vi "CMI Sync V3 Set Tigger.vi"(8 "error in":errorcluster, 9 "Trigger input logic (5V)":T1=enum."TTL 5V", 10 "Trigger mode (Auto)":T2=enum."Auto (continuous)", 11 "session in":T3={"VISA"="", "baud rate [bd/s]"=115200, "source"=enum."Auto", "hv range"=enum."1kV", "fsrc is fixed"=FALSE, "fsrc [Hz]"=10000000.0, "freq integ [s]"=1.0, "freq filter"=5, "trig level"=enum."TTL 5V", "chn1 mode"=enum."Source divider", "chn1 level"=enum."Positive 5V", "chn2 mode"=enum."Source divider", "chn2 level"=enum."Positive 5V", "chn2 div"=1, "chn3 mode"=enum."Chn 1 Active", "chn3 level"=enum."Positive 5V", "chn1 div entry"=enum."Calculate nearest divisor from measured fx", "chn1 dev limit [%]"=1.0, "chn1 check dev"=FALSE} {"chn2 div" min=1 max=100000000 step=1; "fsrc [Hz]" format="%_8p"}) -> (0 "error out":errorcluster, 3 "session out":T3={"VISA"="", "baud rate [bd/s]"=115200, "source"=enum."Auto", "hv range"=enum."1kV", "fsrc is fixed"=FALSE, "fsrc [Hz]"=10000000.0, "freq integ [s]"=1.0, "freq filter"=5, "trig level"=enum."TTL 5V", "chn1 mode"=enum."Source divider", "chn1 level"=enum."Positive 5V", "chn2 mode"=enum."Source divider", "chn2 level"=enum."Positive 5V", "chn2 div"=1, "chn3 mode"=enum."Chn 1 Active", "chn3 level"=enum."Positive 5V", "chn1 div entry"=enum."Calculate nearest divisor from measured fx", "chn1 dev limit [%]"=1.0, "chn1 check dev"=FALSE} {"chn2 div" min=1 max=100000000 step=1; "fsrc [Hz]" format="%_8p"})   [LabVIEW 2020, in "AWG.lvlib" / "CMI Sync Unit V3.lvlib"]
doc: "Sets trigger source and parameters."
uses:
  CMI Sync Unit V3.lvlib
  CMI Sync V3 session.ctl
  CMI Sync V3 Reference Clock Source.ctl
  CMI Sync V3 HV input Range.ctl
  CMI Sync V3 Trigger Input Level.ctl
  CMI Sync V3 Channel 1 Mode.ctl
  CMI Sync V3 Channel Output Levels.ctl
  CMI Sync V3 Channel 2 Mode.ctl
  CMI Sync V3 Channel 3 Mode.ctl
  CMI Sync V3 Channel 1 Divisor Entry Mode.ctl
  CMI Sync V3 Trigger Mode.ctl
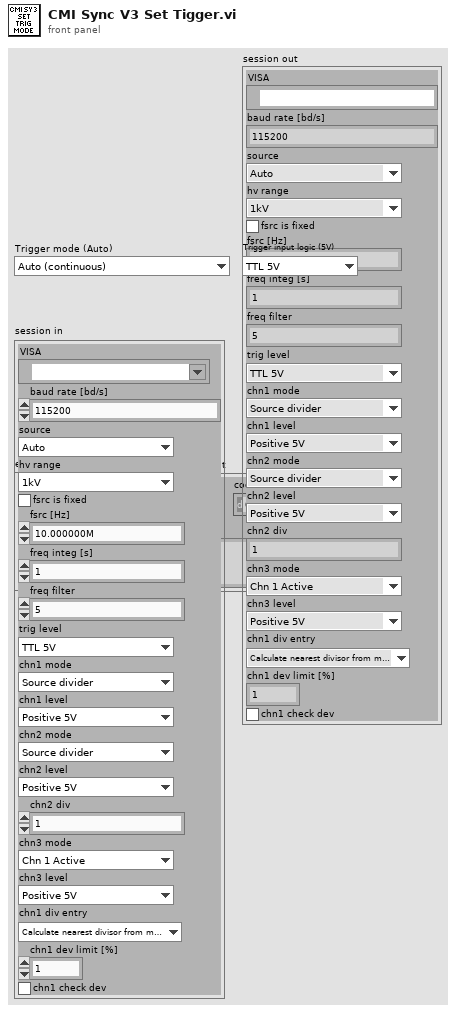
[diagram p1: front panel]
types:
  T1 = typedef "AWG.lvlib/CMI Sync Unit V3.lvlib/CMI Sync V3 Trigger Input Level.ctl" = enum16{"LVCMOS 3V3", "TTL 5V"}
  T2 = typedef "AWG.lvlib/CMI Sync Unit V3.lvlib/CMI Sync V3 Trigger Mode.ctl" = enum16{"Hold", "Auto (continuous)", "Gate positive", "Gate negative", "Rising edge", "Falling edge", "Bus (*TRG)", "Manual (button)"}
  T3 = typedef "AWG.lvlib/CMI Sync Unit V3.lvlib/CMI Sync V3 session.ctl" = cluster{"VISA":refnum<visa-resource-name>, "baud rate [bd/s]":i32, "source":T4, "hv range":T5, "fsrc is fixed":bool, "fsrc [Hz]":dbl, "freq integ [s]":dbl, "freq filter":i32, "trig level":T1, "chn1 mode":T6, "chn1 level":T7, "chn2 mode":T8, "chn2 level":T7, "chn2 div":i32, "chn3 mode":T9, "chn3 level":T7, "chn1 div entry":T10, "chn1 dev limit [%]":dbl, "chn1 check dev":bool}
  T4 = typedef "AWG.lvlib/CMI Sync Unit V3.lvlib/CMI Sync V3 Reference Clock Source.ctl" = enum16{"Auto", "Internal", "Logic", "Sine", "HV"}
  T5 = typedef "AWG.lvlib/CMI Sync Unit V3.lvlib/CMI Sync V3 HV input Range.ctl" = enum16{"10V", "60V", "250V", "1kV"}
  T6 = typedef "AWG.lvlib/CMI Sync Unit V3.lvlib/CMI Sync V3 Channel 1 Mode.ctl" = enum16{"Source divider", "DDS absolute", "DDS ratio", "DDS ratio M/N"}
  T7 = typedef "AWG.lvlib/CMI Sync Unit V3.lvlib/CMI Sync V3 Channel Output Levels.ctl" = enum16{"Positive 3V3", "Negative 3V3", "Positive 5V", "Negative 5V"}
  T8 = typedef "AWG.lvlib/CMI Sync Unit V3.lvlib/CMI Sync V3 Channel 2 Mode.ctl" = enum16{"Source divider", "Chn 1 divide"}
  T9 = typedef "AWG.lvlib/CMI Sync Unit V3.lvlib/CMI Sync V3 Channel 3 Mode.ctl" = enum16{"Chn 1 Active", "Chn 2 Active", "Chn 1 Trigger", "Chn 2 Trigger", "Gate", "PPS", "10MHz"}
  T10 = typedef "AWG.lvlib/CMI Sync Unit V3.lvlib/CMI Sync V3 Channel 1 Divisor Entry Mode.ctl" = enum16{"Set divisor directly", "Calculate nearest divisor from measured fx"}
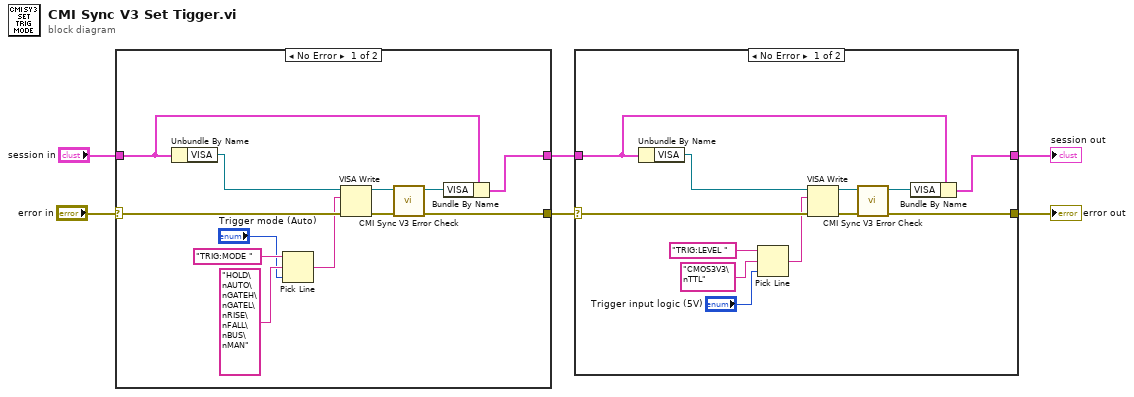
[diagram p0: block diagram]
diagram:
  n1 = case shown="No Error" "error in" {
    selector: "error in" -> [w10 w20]
    tunnel: "session in" -> [w18 w19]
    tunnel: [w17 w19] -> w3
    tunnel: [w12 w20] -> w4
    frame No Error {
      n2 = Unbundle By Name(w18) -> ("VISA"=w16:refnum<visa-resource-name>)
      n3 = Pick Line(string ("")="TRIG:MODE " ("format string"), multi-line string="HOLD\nAUTO\nGATEH\nGATEL\nRISE\nFALL\nBUS\nMAN", line index="Trigger mode (Auto)") -> (output string=w9:string)
      n4 = VISA Write(VISA resource name=w16, write buffer=w9, error in (no error)=w10) -> (VISA resource name out=w14:refnum<visa-resource-name>, error out=w15:errorcluster)  [unwired: 1 out]
      n5 = call "CMI Sync V3 Error Check.vi"("error in"=w15, "VISA in"=w14) -> ("error out"=w12:errorcluster, "VISA out"=w13:refnum<visa-resource-name>)  [unwired: 7 in, 1 out]
      n6 = Bundle By Name(cluster=w18, "VISA"=w13) -> (w17:T3)
    }
    frame Error {
    }
  }
  n7 = case shown="No Error" w4 {
    selector: w4 -> [w25 w34]
    tunnel: w3 -> [w32 w33]
    tunnel: [w31 w33] -> w1
    tunnel: [w26 w34] -> w2
    frame No Error {
      n8 = Unbundle By Name(w32) -> ("VISA"=w30:refnum<visa-resource-name>)
      n9 = Pick Line(string ("")="TRIG:LEVEL " ("format string"), multi-line string="CMOS3V3\nTTL", line index="Trigger input logic (5V)") -> (output string=w21:string)
      n10 = VISA Write(VISA resource name=w30, write buffer=w21, error in (no error)=w25) -> (VISA resource name out=w28:refnum<visa-resource-name>, error out=w29:errorcluster)  [unwired: 1 out]
      n11 = call "CMI Sync V3 Error Check.vi"("error in"=w29, "VISA in"=w28) -> ("error out"=w26:errorcluster, "VISA out"=w27:refnum<visa-resource-name>)  [unwired: 7 in, 1 out]
      n12 = Bundle By Name(cluster=w32, "VISA"=w27) -> (w31:T3)
    }
    frame Error {
    }
  }
  "error out" <- w2
  "session out" <- w1
